vi "Main gScript UI.vi"() -> ()   [LabVIEW 2026]
uses:
  UI typedefs/gScript Controller Status.ctl
  gScript Interpreter/Type Definitions/Main Memory.ctl
  gScript Interpreter/Type Definitions/Memory Cell.ctl
  gScript Interpreter/Type Definitions/Memory Cell Type Enum.ctl
  gScript Interpreter/Type Definitions/Stack Frame.ctl
  gScript Interpreter/Type Definitions/Variable Table.ctl
  gScript Interpreter/Type Definitions/Variable.ctl
  Shared Components/Gantry Class/Type Definitions/Virtual Modes.ctl
  UI typedefs/gScript Controller Commands.ctl
  Shared Components/Gantry Class/Gantry.lvclass
  <instrlib>/Aerotech Automation1/Aerotech.Automation1.DotNet.dll
  gScript Interpreter/gScript Interpreter.lvclass
  Application Utilities/Console Log/Console Log.lvclass
  C:/Users/User/Desktop/pixel-gantry-control/Gantry/A3200/Bin/Aerotech.A3200.dll
  A3200/Bin/Aerotech.A3200.dll
  <instrlib>/Aerotech Automation1/Aerotech Automation1.lvlib
panel:
  out "Aerotech controller Ref":T2
  in  "Virtual Mode":bool=TRUE
  out "Command History idx":i32
  out "Abort Async Request":bool=TRUE
  in  "Tab Control":enum32{"Control", "Memory", "Command History"}(tab)
  in  "Load Project":bool
  out "Line Indicator":string
  out "version":string
  out "Script Path":path
  in  "ESTOP":bool
  in  "Execute":bool
  in  "Command Input":string
  out "Status":T3
  in  "Abort Script":bool
  in  "EXIT":bool
  in  "Pause Script":bool
  in  "Run Script":bool
  in  "Load Script":bool
  in  "Script Input":string
  in  "Save Script":bool
  out "Console":string
  in  "Variable Table":T4[](array[typedef])
  in  "Main Memory":T9
  in  "Memory Size":i32=256
  out "Command History":string[](array[string])
  # "Documentation:  https://github.com/CUASAS/pixel-gantry-control/blob/master/Gantry/gScript%20Application/gScript%20Documentation.md"
  # "Command Input >"
  # "Stack Index"
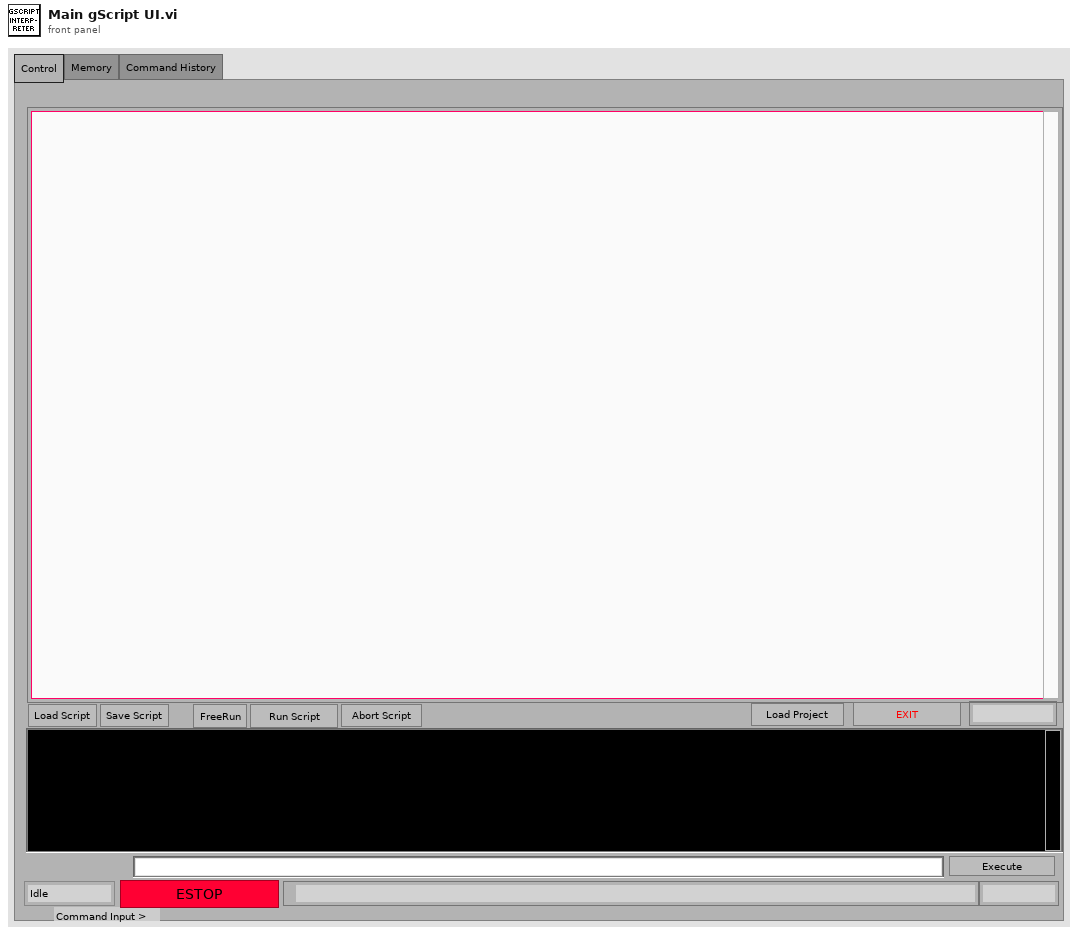
[diagram p1: front panel]
types:
  T1 = typedef "Virtual Modes.ctl" = enum16{"Nonvirtual", "Virtual"}
  T2 = cluster{"Controller Ref":variant, "Virtual Mode":T1}
  T3 = typedef "gScript Controller Status.ctl" = enum16{"Idle", "Running", "Paused"}
  T4 = typedef "Stack Frame.ctl" = cluster{"Variable Table":T5, "Return Pointer":i32, "Return Bindings":string[]}
  T5 = typedef "Variable Table.ctl" = T6[]
  T6 = typedef "Variable.ctl" = cluster{"Variable Name":string, "Memory Cell":T7}
  T7 = typedef "Memory Cell.ctl" = cluster{"type":T8, "x":dbl, "y":dbl, "z":dbl, "w":dbl}
  T8 = typedef "Memory Cell Type Enum.ctl" = enum16{"integer", "float", "vector", "rotation"}
  T9 = typedef "Main Memory.ctl" = T7[]
  T10 = typedef "gScript Controller Commands.ctl" = enum16{"Initialize", "Run Script", "Abort Script", "Exit", "Load Script", "Save Script", "Run Command", "ESTOP Pressed", "Quicksave", "Load Project"}
  T11 = enum8{"Enabled", "Disabled", "Disabled and Grayed Out"}
  T12 = cluster{"Shift":bool, "Ctrl":bool, "Alt":bool, "Cmd":bool, "Opt":bool}
  T13 = enum16{"open", "replace", "create", "open or create", "replace or create", "replace or create with confirmation"}
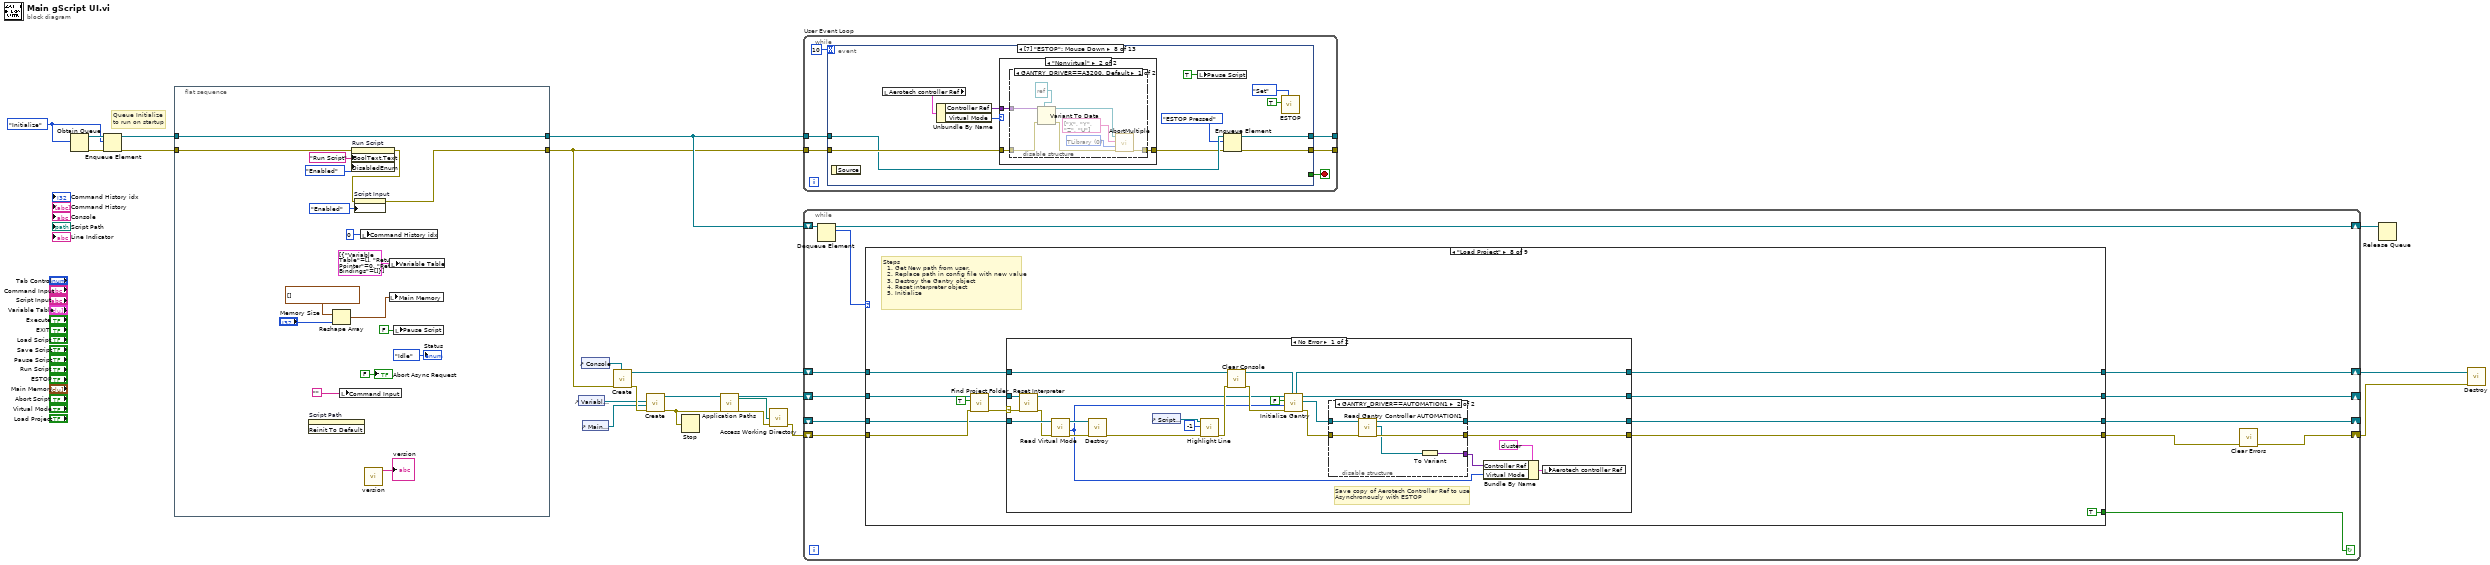
[diagram p0: block diagram]
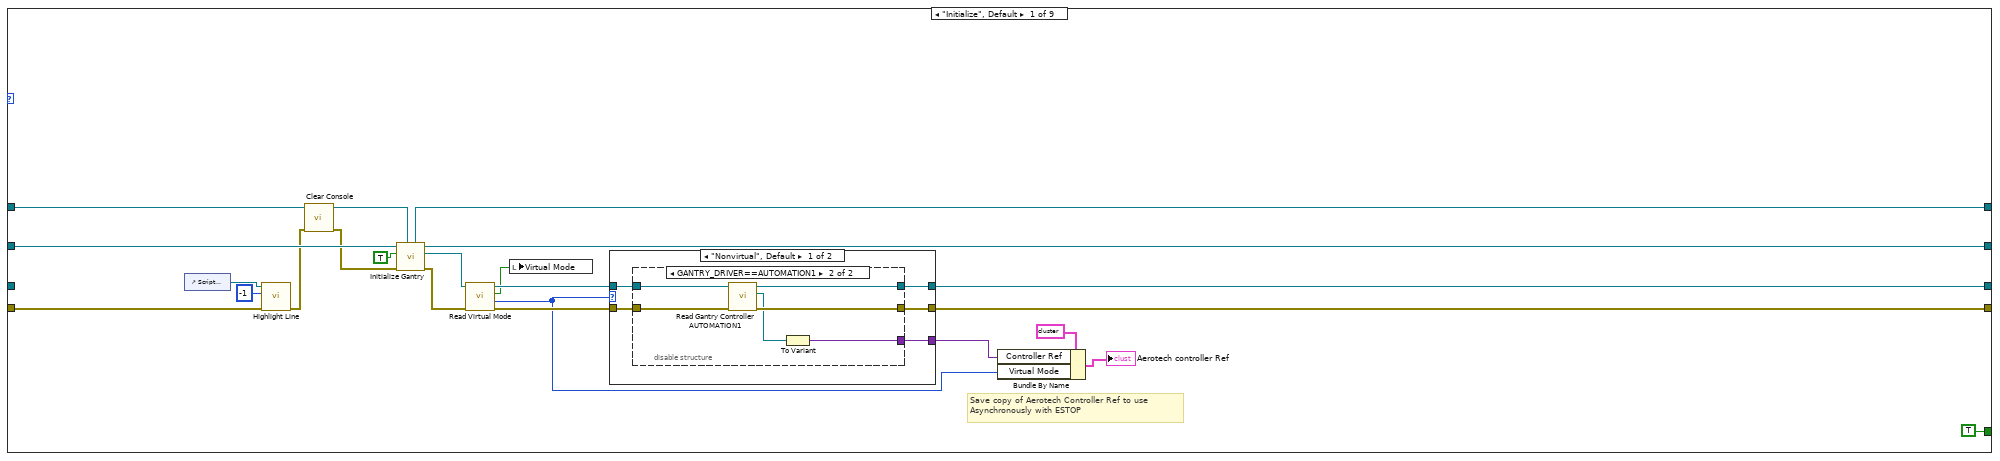
[diagram p2: hidden frame]
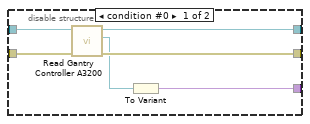
[diagram p3: hidden frame]
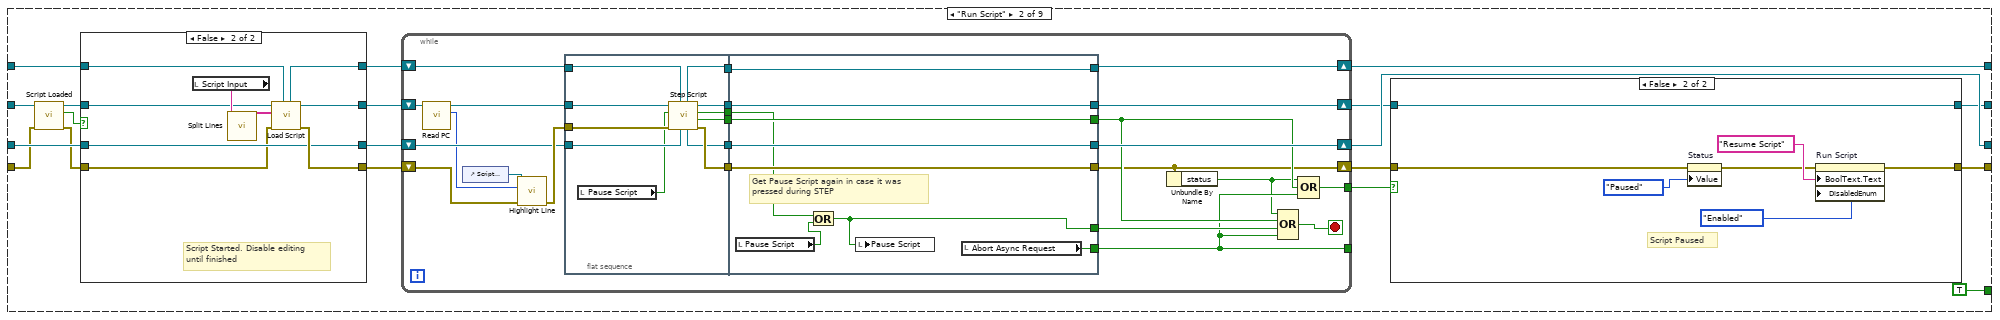
[diagram p5: hidden frame]
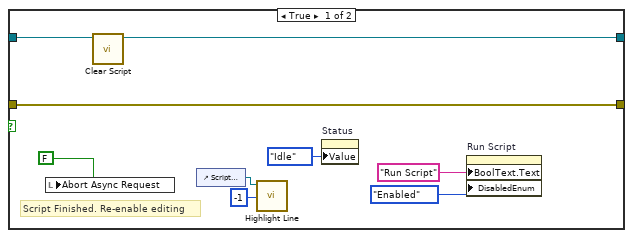
[diagram p7: hidden frame]
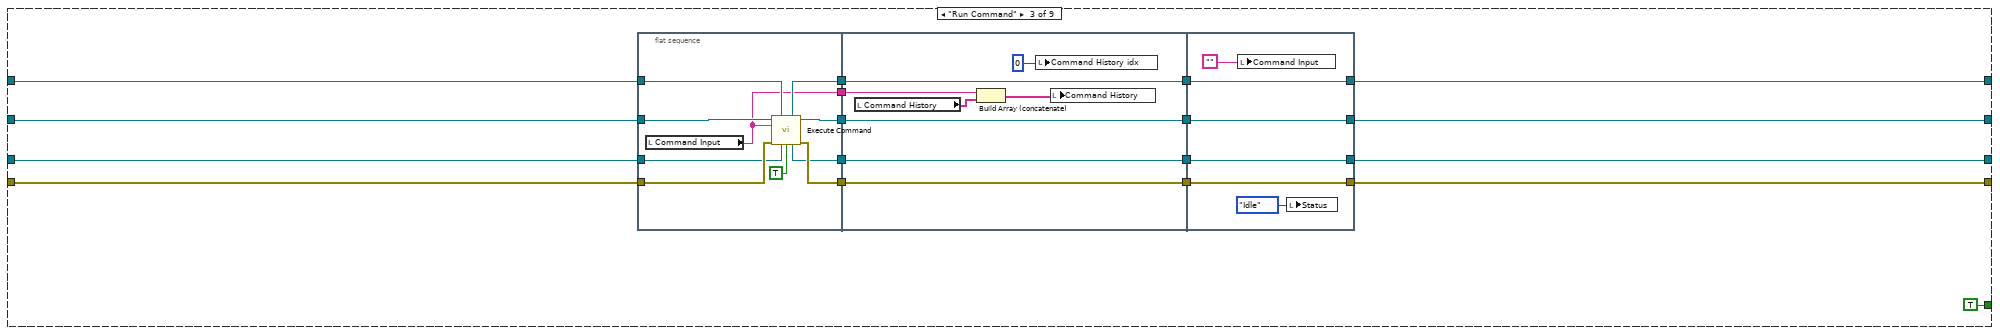
[diagram p8: hidden frame]
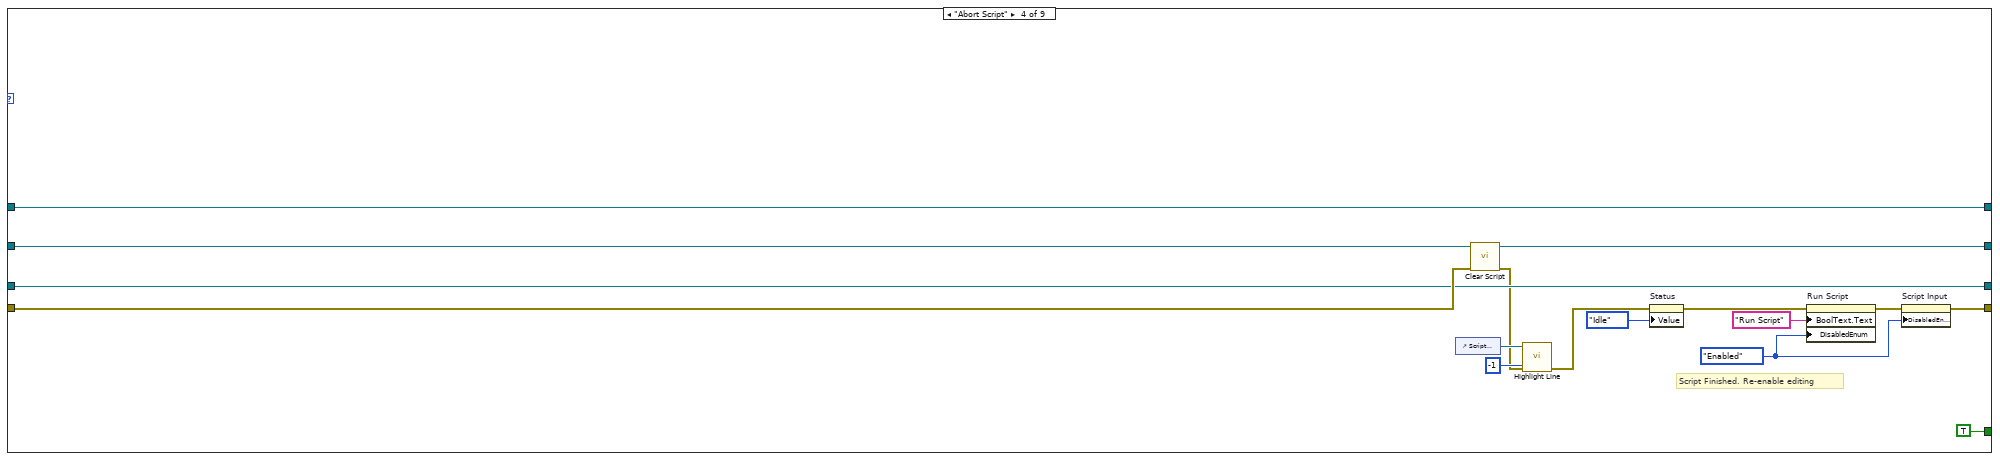
[diagram p9: hidden frame]
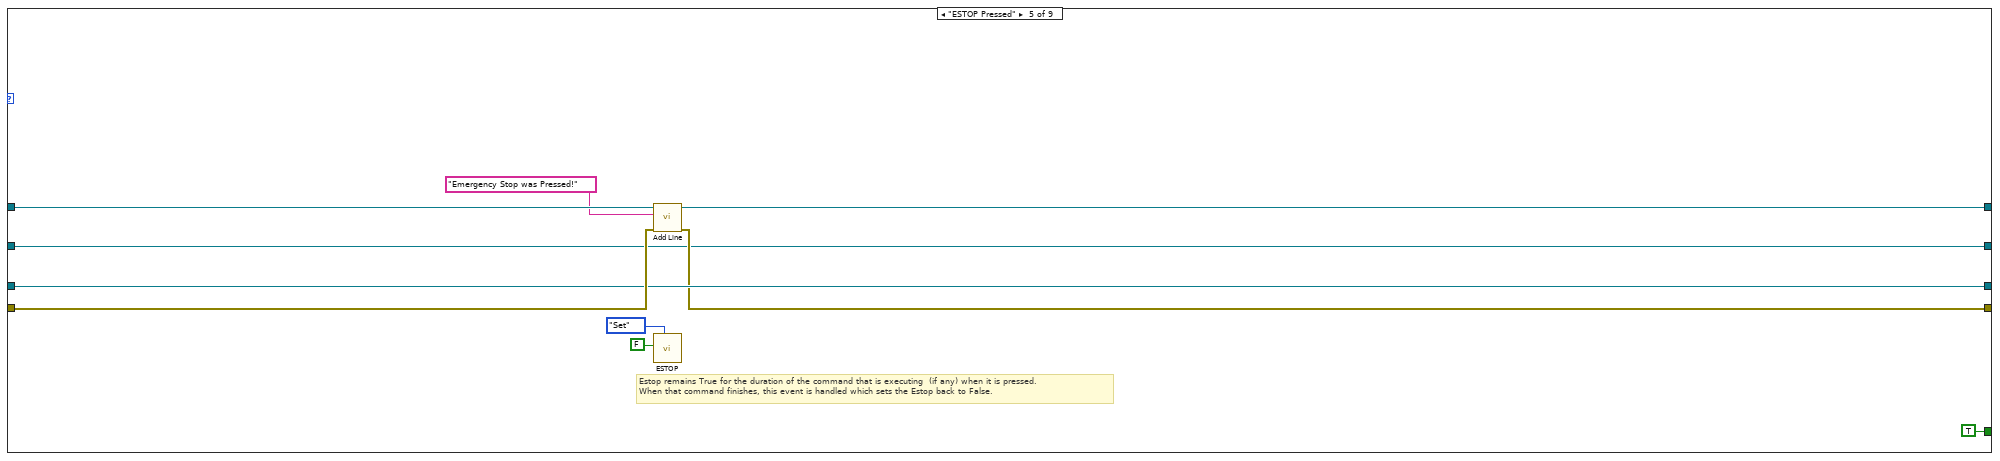
[diagram p10: hidden frame]
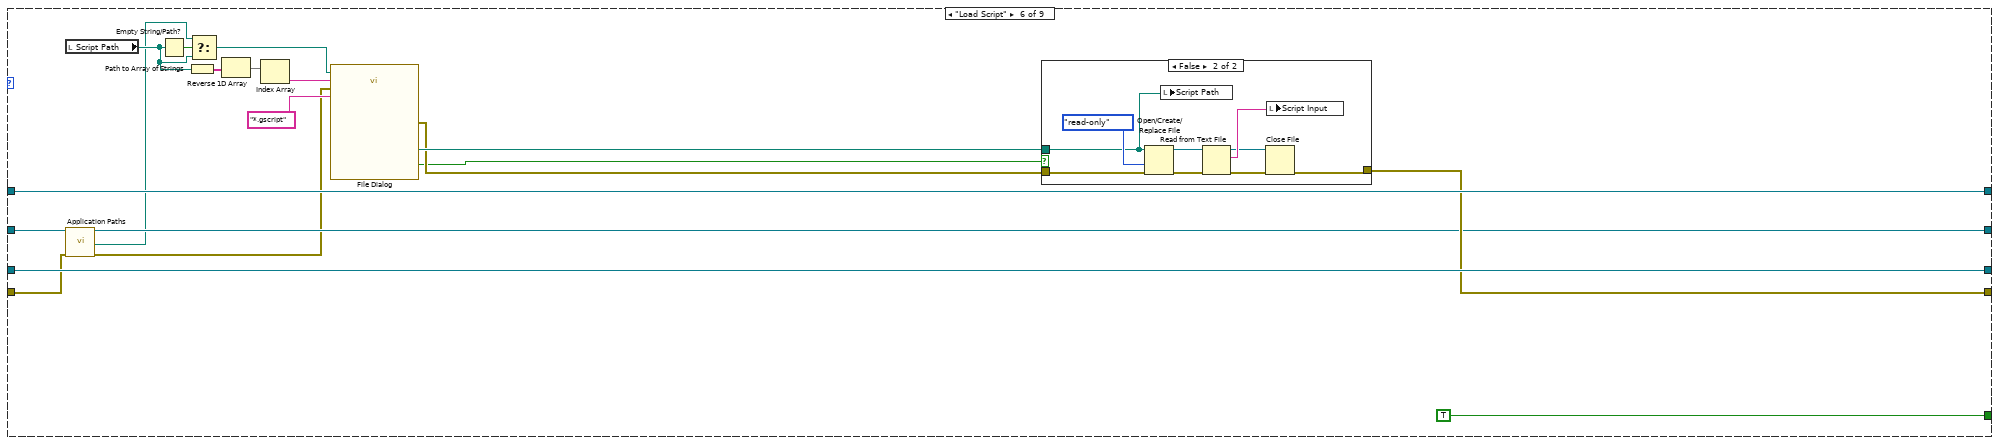
[diagram p11: hidden frame]
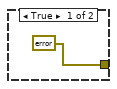
[diagram p12: hidden frame]
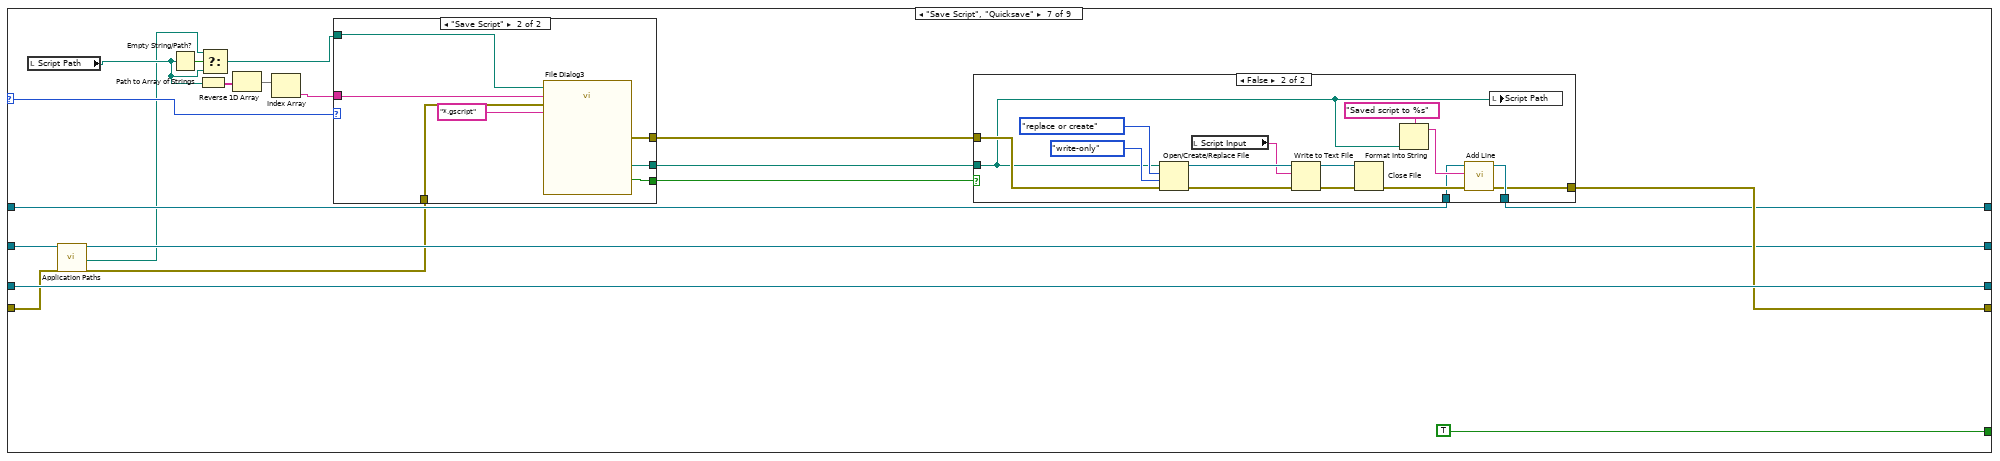
[diagram p13: hidden frame]
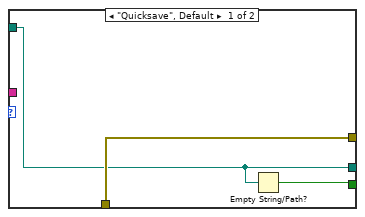
[diagram p14: hidden frame]
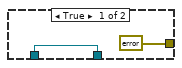
[diagram p15: hidden frame]
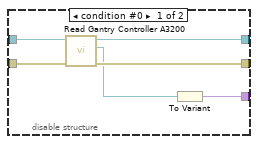
[diagram p16: hidden frame]
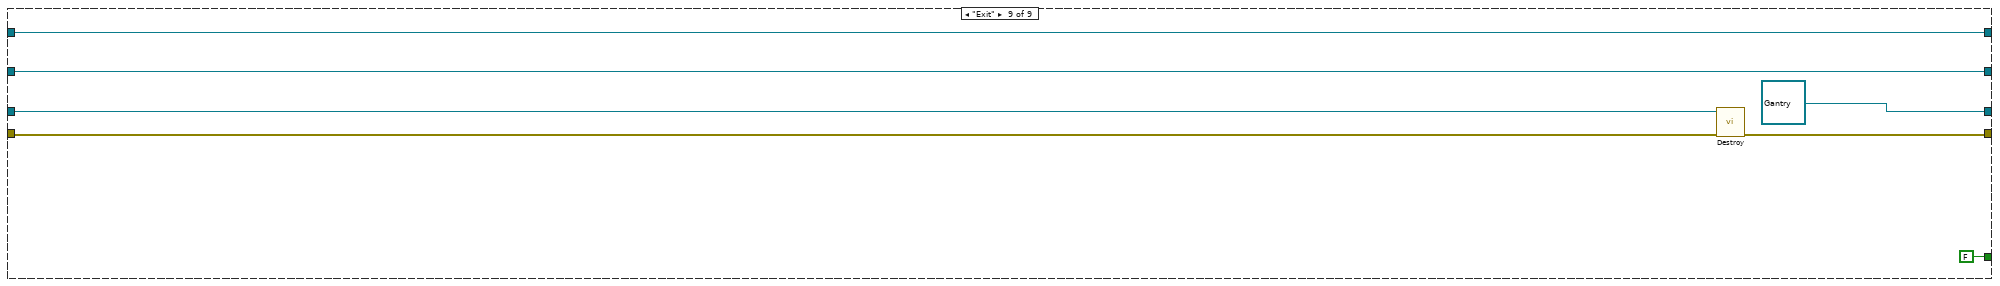
[diagram p18: hidden frame]
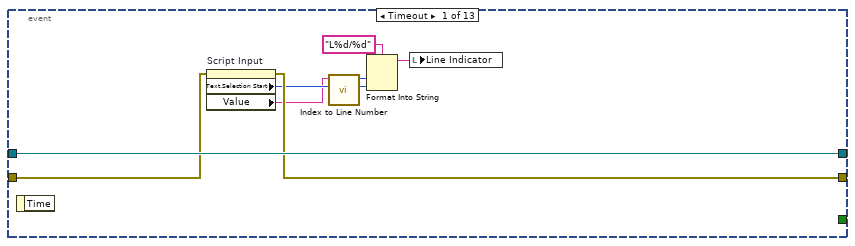
[diagram p19: hidden frame]
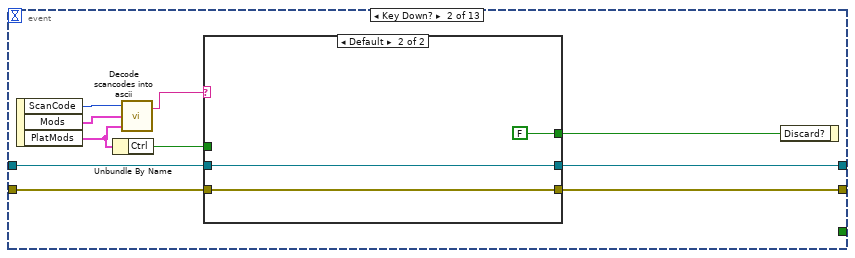
[diagram p20: hidden frame]
diagram:
  w18 = gScript_Controller_Commands."Initialize"
  # "Queue Initialize \nto run on startup"
  n1 = Obtain Queue(element data type=w18) -> (queue out=w20:refnum<queue>, error out=w19:errorcluster)  [unwired: 4 in, 1 out]
  n2 = Enqueue Element(queue=w20, element=w18, error in (no error)=w19) -> (queue out=w14:refnum<queue>, error out=w12:errorcluster)  [unwired: 1 in, 1 out]
  n3 = flat-sequence {
    tunnel: w14 -> [w38]
    tunnel: [w38] -> w13
    tunnel: w12 -> [w34]
    tunnel: [w31] -> w11
    frame #0 {
      n4 = invoke on="Script Path" class="Path" method="Reinit To Default"() -> ()  [unwired: 3 in, 3 out]
      n5 = Reshape Array(T7[] [] ("Main Memory"), "Memory Size") -> (w26:T7[])
      n6 = local write "Command Input"("") -> ()
      n7 = property on="Run Script" class="Bool (strict)"(error in=w34, "BoolText.Text"="Run Script" ("Boolean Text.Text"), "DisabledEnum"=T11."Enabled" ("Disabled")) -> (error out=w32:errorcluster)  [unwired: 1 in, 1 out]
      n8 = property on="Script Input" class="Str"(error in=w32, "DisabledEnum"=T11."Enabled" ("Disabled")) -> (error out=w31:errorcluster)  [unwired: 1 in, 1 out]
      n9 = local write "Command History idx"(0 ("Command History idx")) -> ()
      n10 = call "version.vi"() -> ("Version"=→"version":string)  [unwired: 3 in]
      n11 = local write "Main Memory"(w26) -> ()
      n12 = local write "Variable Table"(T4[] [{"Variable Table"=[], "Return Pointer"=0, "Return Bindings"=[]}] ("Variable Table")) -> ()
      n13 = local write "Pause Script"(FALSE ("Pause Script")) -> ()
      "Status" <- gScript_Controller_Status."Idle" ("Status")
      "Abort Async Request" <- FALSE ("Abort Requested")
    }
  }
  n14 = control-ref of="Variable Table"() -> (w7:refnum<vi>)
  n15 = control-ref of="Console"() -> (w21:refnum<vi>)
  n16 = control-ref of="Main Memory"() -> (w9:refnum<vi>)
  n17 = call "Create.vi"("Console"=w21, "error in"=w11) -> ("error out"=w15:errorcluster, "Console Log out"=w17:refnum<class "Console Log.lvclass">)  [unwired: 8 in]
  n18 = call "Create.vi"("error in (no error)"=w15, "Main Memory Ref"=w9, "Variable Table Ref"=w7) -> ("error out"=w1:errorcluster, "gScript Interpreter out"=w6:refnum<class "gScript Interpreter.lvclass">)  [unwired: 7 in]
  n19 = Stop(stop? (T)=w1) -> ()
  n20 = call "Application Paths.vi"("gScript Interpreter in"=w6, "error in (no error)"=w1) -> ("gScript Interpreter out"=w3:refnum<class "gScript Interpreter.lvclass">, "Project Path"=w2:path, "error out"=w5:errorcluster)  [unwired: 12 in, 3 out]
  n21 = call "Access Working Directory.vi"("error in (no error)"=w5, "Set Directory"=w2) -> ("error out"=w4:errorcluster)  [unwired: 2 in, 1 out]
  n22 = while "User Event Loop" {
    tunnel: w13 -> [w39]
    tunnel: [w42] -> _
    tunnel: w11 -> [w41]
    tunnel: [w40] -> _
    stop <- w43 stop-if-true
    n23 = event shown="[7] \"ESTOP\": Mouse Down" {
      selector: _ -> [_ _ _ _ _ _ _ _ _ _ _ _ _]
      dyn-events: _ -> [_ _ _ _ _ _ _ _ _ _ _ _ _]
      timeout: 10 -> [_ _ _ _ _ _ _ _ _ _ _ _ _]
      tunnel: [_ _ _ _ _ _ _ _ _ _ TRUE ("T button?") _ TRUE ("T button?")] -> w43
      tunnel: w39 -> [w53 w58 w85 w122 w138 w180 w202 w221 w247 w260 w272 w286 w292]
      tunnel: [w53 w56 w83 w120 w136 w177 w201 w218 w244 w258 w277 w284 w290] -> w42
      tunnel: w41 -> [w52 w57 w84 w121 w137 w179 w200 w223 w246 w259 w271 w285 w291]
      tunnel: [w51 w55 w82 w119 w135 w178 w199 w219 w243 w257 w276 w283 w289] -> w40
      event Timeout {
        n24 = event-data() -> ()  [unwired: 1 in, 1 out]
        n25 = property on="Script Input" class="Str"(error in=w52) -> (error out=w51:errorcluster, "Text.Selection Start"=w50:u32, "Value"=w49:string)  [unwired: 1 in, 1 out]
        n26 = call "Index to Line Number.vi"("Index"=w50, "Text"=w49) -> ("Line Count"=w45:u32, "Line Number"=w47:u32)  [unwired: 8 in]
        n27 = Format Into String(format string="L%d/%d", w47, w45) -> (resulting string=w46:string)  [unwired: 2 in, 1 out]
        n28 = local write "Line Indicator"(w46) -> ()
      }
      event Key Down? {
        n29 = event-data() -> ("ScanCode"=w63:i16, "Mods"=w61:cluster{"Num Pad":bool, "Menu Key":bool}, "PlatMods"=w60:T12)  [unwired: 1 in]
        n30 = Unbundle By Name(w60) -> ("Ctrl"=w59:bool)
        n31 = call "Decode scancodes into ascii.vi"("PlatMods"=w60, "Mods"=w61, "ScanCode"=w63) -> ("String"=w62:string)  [unwired: 1 out]
        n32 = case shown="Default" w62 {
          tunnel: w59 -> [w69 _]
          tunnel: w58 -> [w66 w81]
          tunnel: w57 -> [w68 w80]
          tunnel: [w65 w81] -> w56
          tunnel: [w67 w80] -> w55
          tunnel: [w64 FALSE] -> w54
          frame "s" {
            n33 = case shown="False" w69 {
              tunnel: w68 -> [w72 w77]
              tunnel: [w72 w76] -> w67
              tunnel: w66 -> [w71 w78]
              tunnel: [w71 w75] -> w65
              tunnel: [FALSE TRUE] -> w64
              frame False {
              }
              frame True {
                n34 = Enqueue Element(queue=w78, element=gScript_Controller_Commands."Quicksave", error in (no error)=w77) -> (queue out=w75:refnum<queue>, error out=w76:errorcluster)  [unwired: 1 in, 1 out]
              }
            }
          }
          frame Default {
          }
        }
        n35 = event-data("Discard?"=w54) -> ()  [unwired: 1 in, 1 out]
      }
      event "Script Input": Key Down? {
        n36 = event-data() -> ("ScanCode"=w90:i16, "Mods"=w89:cluster{"Num Pad":bool, "Menu Key":bool}, "PlatMods"=w88:T12)  [unwired: 1 in]
        n37 = local read "Status"() -> (w92:T3)
        n38 = call "Decode scancodes into ascii.vi"("PlatMods"=w88, "Mods"=w89, "ScanCode"=w90) -> ("Numeric"=w86:i16, "String"=w87:string)
        n39 = case shown="\"Idle\", Default" w92 {
          tunnel: [w98 TRUE] -> w91
          tunnel: w87 -> [w97 _]
          tunnel: w86 -> [_ _]
          tunnel: w85 -> [w96 w116]
          tunnel: w84 -> [w94 w115]
          tunnel: [w95 w116] -> w83
          tunnel: [w93 w115] -> w82
          frame "Idle", Default {
            n40 = case shown="\"tab\"" w97 {
              tunnel: [TRUE FALSE] -> w98
              tunnel: w96 -> [w99 w113]
              tunnel: [w99 w113] -> w95
              tunnel: w94 -> [w107 w112]
              tunnel: [w104 w112] -> w93
              frame "tab" {
                # "four spaces"
                n41 = control-ref of="Script Input"() -> (w110:refnum<vi>)
                n42 = property class="Str"(reference=w110, error in=w107) -> (reference out=w108:refnum<vi>, error out=w106:errorcluster, "Text.Selection End"=w102:u32, "Value"=w109:string)
                n43 = Add(x=w102, y=u32 4) -> (x+y=w100:u32)
                n44 = call "Insert Text.vi"("Insert String"="    ", "Insert Position"=w102, "Source String"=w109) -> ("Output String"=w105:string)
                n45 = property class="Str"(reference=w108, error in=w106, "Value"=w105, "Text.Selection End"=w100, "Text.Selection Start"=w100) -> (error out=w104:errorcluster)  [unwired: 1 out]
              }
              frame Default {
              }
            }
          }
          frame "Running", "Paused" {
            # "Disable editing the script while it is running"
          }
        }
        n46 = event-data("Discard?"=w91) -> ()  [unwired: 1 in, 1 out]
      }
      event "Execute": Value Change {
        n47 = event-data() -> ("NewVal"=w118:bool)  [unwired: 1 in]
        n48 = case shown="True" w118 {
          tunnel: w122 -> [w123 w130]
          tunnel: w121 -> [w124 w127]
          tunnel: [w123 w129] -> w120
          tunnel: [w124 w126] -> w119
          frame False {
          }
          frame True {
            n49 = Enqueue Element(queue=w130, element=gScript_Controller_Commands."Run Command", error in (no error)=w127) -> (queue out=w129:refnum<queue>, error out=w126:errorcluster)  [unwired: 1 in, 1 out]
            n50 = local write "Status"(gScript_Controller_Status."Running" ("Status")) -> ()
          }
        }
      }
      event "Command Input": Key Down {
        n51 = event-data() -> ("ScanCode"=w134:i16, "Mods"=w133:cluster{"Num Pad":bool, "Menu Key":bool}, "PlatMods"=w132:T12)  [unwired: 1 in]
        n52 = call "Decode scancodes into ascii.vi"("PlatMods"=w132, "Mods"=w133, "ScanCode"=w134) -> ("String"=w131:string)  [unwired: 1 out]
        n53 = case shown="\"UP\"" w131 {
          tunnel: w138 -> [w144 w153 w154 w163]
          tunnel: w137 -> [w143 w152 w155 w161]
          tunnel: [w144 w153 w154 w162] -> w136
          tunnel: [w143 w152 w155 w160] -> w135
          frame "UP" {
            n54 = local read "Command History idx"() -> (w140:i32)
            n55 = local read "Command History"() -> (w142:string[])
            n56 = Index Array(array=w142, index=w140) -> (element=w141:string)
            n57 = Increment(x=w140) -> (x+1=w139:i32)
            n58 = local write "Command Input"(w141) -> ()
            n59 = local write "Command History idx"(w139) -> ()
          }
          frame "DOWN" {
            n60 = local read "Command History idx"() -> (w149:i32)
            n61 = local read "Command History"() -> (w150:string[])
            n62 = Decrement(x=w149) -> (x-1=w148:i32)
            n63 = In Range and Coerce(upper limit=1000 ("lower limit"), x=w148, lower limit=0) -> (coerced(x)=w147:i32)  [unwired: 1 out]
            n64 = Index Array(array=w150, index=w147) -> (element=w146:string)
            n65 = local write "Command Input"(w146) -> ()
            n66 = local write "Command History idx"(w147) -> ()
          }
          frame Default {
          }
          frame "Enter" {
            n67 = flat-sequence {
              tunnel: w163 -> [w166]
              tunnel: w161 -> [w167]
              tunnel: [w167] -> w159
              tunnel: [w166] -> w158
              tunnel: w159 -> [w168]
              tunnel: w158 -> [w170]
              tunnel: [w172] -> w157
              tunnel: [w171] -> w156
              tunnel: [w174] -> w160
              tunnel: [w175] -> w162
              tunnel: w157 -> [w175]
              tunnel: w156 -> [w174]
              frame #0 {
                # "Does not work without this pause"
                n68 = local write "Status"(gScript_Controller_Status."Running" ("Status")) -> ()
                n69 = Wait (ms)(milliseconds to wait=u32 100) -> ()  [unwired: 1 out]
              }
              frame #1 {
                n70 = Enqueue Element(queue=w170, element=gScript_Controller_Commands."Run Command", error in (no error)=w168) -> (queue out=w172:refnum<queue>, error out=w171:errorcluster)  [unwired: 1 in, 1 out]
              }
              frame #2 {
                n71 = property on="Command Input" class="Str"("Key Focus"=TRUE) -> ()  [unwired: 2 in, 2 out]
              }
            }
          }
        }
      }
      event "Run Script": Mouse Up {
        n72 = event-data() -> ()  [unwired: 1 in, 1 out]
        n73 = local read "Status"() -> (w176:T3)
        n74 = case shown="\"Idle\"" w176 {
          tunnel: w180 -> [w182 w190 w197]
          tunnel: w179 -> [w181 w189 w196]
          tunnel: [w181 w188 w193] -> w178
          tunnel: [w182 w187 w194] -> w177
          frame "Running" {
          }
          frame "Idle" {
            n75 = Enqueue Element(queue=w190, element=gScript_Controller_Commands."Run Script", error in (no error)=w189) -> (queue out=w187:refnum<queue>, error out=w188:errorcluster)  [unwired: 1 in, 1 out]
            n76 = property on="Run Script" class="Bool (strict)"("BoolText.Text"="Running" ("Boolean Text.Text"), "DisabledEnum"=T11."Disabled and Grayed Out" ("Disabled")) -> ()  [unwired: 2 in, 2 out]
            n77 = local write "Status"(gScript_Controller_Status."Running" ("Status")) -> ()
          }
          frame "Paused" {
            n78 = Enqueue Element(queue=w197, element=gScript_Controller_Commands."Run Script", error in (no error)=w196) -> (queue out=w194:refnum<queue>, error out=w193:errorcluster)  [unwired: 1 in, 1 out]
            n79 = property on="Run Script" class="Bool (strict)"("BoolText.Text"="Running" ("Boolean Text.Text"), "DisabledEnum"=T11."Disabled and Grayed Out" ("Disabled")) -> ()  [unwired: 2 in, 2 out]
            n80 = local write "Status"(gScript_Controller_Status."Running" ("Status")) -> ()
          }
        }
      }
      event "Abort Script": Mouse Up {
        n81 = event-data() -> ()  [unwired: 1 in, 1 out]
        n82 = local read "Status"() -> (w203:T3)
        n83 = case shown="\"Idle\", \"Paused\"" w203 {
          tunnel: w202 -> [w205 w210]
          tunnel: [w205 w209] -> w201
          tunnel: w200 -> [w204 w208]
          tunnel: [w204 w207] -> w199
          frame "Running" {
            n84 = local write "Abort Async Request"(TRUE ("Abort Requested")) -> ()
          }
          frame "Idle", "Paused" {
            n85 = Enqueue Element(queue=w210, element=gScript_Controller_Commands."Abort Script", error in (no error)=w208) -> (queue out=w209:refnum<queue>, error out=w207:errorcluster)  [unwired: 1 in, 1 out]
          }
        }
      }
      event "ESTOP": Mouse Down {
        n86 = event-data() -> ()  [unwired: 1 in, 1 out]
        n87 = local read "Aerotech controller Ref"() -> (w214:T2)
        n88 = Unbundle By Name(w214) -> ("Controller Ref"=w213:variant, "Virtual Mode"=w212:T1)
        n89 = case shown="\"Nonvirtual\"" w212 {
          tunnel: w223 -> [w224 w225]
          tunnel: [w224 w227] -> w220
          tunnel: w213 -> [_ w226]
          frame "Virtual" {
          }
          frame "Nonvirtual" {
            n90 = disable-structure shown="GANTRY_DRIVER==A3200, Default" {
              disable-tunnel: [w233 w236] -> w227
              disable-tunnel: w226 -> [w231 w238]
              disable-tunnel: w225 -> [w229 w237]
              frame condition #0 {
                w234 = 0 items=["TLibrary", "T01", "T02", "T03", "T04", "T05", "T06", "T07", "T08", "T09", "T10", "T11", "T12", "T13", "T14", "T15", "T16", "T17", "T18", "T19", "T20", "T21", "T22", "T23", "T24", "T25", "T26", "T27", "T28", "T29", "T30", "T31"] ("taskId")
                n91 = Variant To Data(error in=w229, type=refnum<k24> refnum ("controller out"), Variant=w231) -> (data=w230:refnum<k24>, error out=w228:errorcluster)
                n92 = call "AbortMultiple.vi"("error in (no error)"=w228, "taskId"=w234, "axis names"=string[] ["X", "Y", "Z", "U"], "controller in"=w230) -> ("error out"=w233:errorcluster)  [unwired: 6 in, 1 out]
              }
              frame condition #1 (active) {
                n93 = Variant To Data(error in=w237, type=refnum<k24> refnum ("Controller Refnum out"), Variant=w238) -> (data=w241:refnum<k24>, error out=w240:errorcluster)
                n94 = call <instrlib>:"Abort.vi"("error in (no error)"=w240, "axisNames"=string[] ["X", "Y", "Z", "U"] ("axis names"), "Controller Refnum"=w241) -> ("error out"=w236:errorcluster)  [unwired: 7 in, 1 out]
              }
            }
          }
        }
        n95 = local write "Pause Script"(TRUE ("Pause Script")) -> ()
        n96 = Enqueue Element(queue=w221, element=gScript_Controller_Commands."ESTOP Pressed", error in (no error)=w220) -> (queue out=w218:refnum<queue>, error out=w219:errorcluster)  [unwired: 1 in, 1 out]
        n97 = call "ESTOP.vi"("Get/Set"=enum16{"Get", "Set"}."Set", "Value In"=TRUE) -> ()  [unwired: 9 in, 1 out]
      }
      event "Load Script": Mouse Up {
        n98 = event-data() -> ()  [unwired: 1 in, 1 out]
        n99 = local read "Status"() -> (w245:T3)
        n100 = case shown="\"Idle\", Default" w245 {
          tunnel: w247 -> [w252 w255]
          tunnel: w246 -> [w251 w254]
          tunnel: [w249 w255] -> w244
          tunnel: [w250 w254] -> w243
          frame "Idle", Default {
            n101 = Enqueue Element(queue=w252, element=gScript_Controller_Commands."Load Script", error in (no error)=w251) -> (queue out=w249:refnum<queue>, error out=w250:errorcluster)  [unwired: 1 in, 1 out]
          }
          frame "Running", "Paused" {
            n102 = One Button Dialog(message="Cannot Load while Script is Running or Paused\nAbort or finish running script first.") -> ()  [unwired: 1 in, 1 out]
          }
        }
      }
      event "Save Script": Mouse Up {
        n103 = event-data() -> ()  [unwired: 1 in, 1 out]
        n104 = local read "Status"() -> (w256:T3)
        n105 = case shown="\"Idle\", Default" w256 {
          tunnel: w260 -> [w265 w268]
          tunnel: w259 -> [w264 w267]
          tunnel: [w262 w268] -> w258
          tunnel: [w263 w267] -> w257
          frame "Idle", Default {
            n106 = Enqueue Element(queue=w265, element=gScript_Controller_Commands."Save Script", error in (no error)=w264) -> (queue out=w262:refnum<queue>, error out=w263:errorcluster)  [unwired: 1 in, 1 out]
          }
          frame "Running", "Paused" {
            n107 = One Button Dialog(message="Cannot Save while Script is Running or Paused\nAbort or finish running script first.") -> ()  [unwired: 1 in, 1 out]
          }
        }
      }
      event "EXIT": Mouse Up {
        n108 = event-data() -> ()  [unwired: 1 in, 1 out]
        n109 = local read "Status"() -> (w273:T3)
        n110 = case shown="Default" w273 {
          tunnel: w272 -> [w279 w281]
          tunnel: w271 -> [w278 w280]
          tunnel: [w279 w281] -> w270
          tunnel: [w278 w280] -> w269
          frame Default {
          }
          frame "Running" {
            n111 = local write "Abort Async Request"(TRUE ("Abort Async Request")) -> ()
          }
        }
        n112 = Enqueue Element(queue=w270, element=gScript_Controller_Commands."Exit", error in (no error)=w269) -> (queue out=w277:refnum<queue>, error out=w276:errorcluster)  [unwired: 1 in, 1 out]
      }
      event "Load Project": Mouse Up {
        n113 = event-data() -> ()  [unwired: 1 in, 1 out]
        n114 = Enqueue Element(queue=w286, element=gScript_Controller_Commands."Load Project", error in (no error)=w285) -> (queue out=w284:refnum<queue>, error out=w283:errorcluster)  [unwired: 1 in, 1 out]
      }
      event Panel Close? {
        n115 = event-data() -> ()  [unwired: 1 in, 1 out]
        n116 = Enqueue Element(queue=w292, element=gScript_Controller_Commands."Exit", error in (no error)=w291) -> (queue out=w290:refnum<queue>, error out=w289:errorcluster)  [unwired: 1 in, 1 out]
        n117 = event-data("Discard?"=TRUE) -> ()  [unwired: 1 in, 1 out]
      }
    }
  }
  n118 = while {
    shift-right: [w296] -> w16
    shift-left: w17 -> [w305]
    shift-right: [w299] -> _
    shift-left: w3 -> [w304]
    shift-right: [w302] -> _
    shift-left: _ -> [w303]
    shift-right: [w297] -> w8
    shift-left: w4 -> [w301]
    shift-right: [w298] -> w10
    shift-left: w13 -> [w307]
    stop <- w300 continue-if-true
    n119 = Dequeue Element(queue=w307) -> (queue out=w298:refnum<queue>, element=w306:T10)  [unwired: 2 in, 2 out]
    n120 = case shown="\"Load Project\"" w306 {
      selector: w306 -> [_ _ _ _ _ _ w552 _ _]
      tunnel: w305 -> [w323 w359 w457 w490 w509 w526 w551 w592 w643]
      tunnel: w304 -> [w325 w357 w459 w493 w502 w514 w543 w597 w644]
      tunnel: w303 -> [_ w361 w453 w487 w506 w528 w558 w587 w641]
      tunnel: [w327 w352 w452 w487 w506 w528 w558 w590 refnum<class "Gantry.lvclass"> refnum ("Gantry Out")] -> w302
      tunnel: w301 -> [w326 w355 w455 w492 w507 w512 w541 w595 w642]
      tunnel: [w312 w363 w454 w489 w505 w522 w556 w588 w640] -> w295
      tunnel: [TRUE TRUE TRUE TRUE TRUE TRUE TRUE TRUE FALSE] -> w300
      tunnel: [w318 w364 w456 w490 w503 w526 w550 w591 w643] -> w296
      tunnel: [w319 w350 w458 w491 w502 w513 w542 w589 w644] -> w299
      frame "Initialize", Default {
        # "Save copy of Aerotech Controller Ref to use\nAsynchronously with ESTOP"
        n121 = control-ref of="Script Input"() -> (w329:refnum<vi>)
        n122 = call "Highlight Line.vi"("error in (no error)"=w326, "Line Number"=-1, "String Field In"=w329) -> ("error out"=w321:errorcluster)  [unwired: 7 in, 1 out]
        n123 = call "Clear Console.vi"("error in (no error)"=w321, "Console Log in"=w323) -> ("error out"=w320:errorcluster, "Console Log out"=w322:refnum<class "Console Log.lvclass">)  [unwired: 8 in]
        n124 = call "Initialize Gantry.vi"("Console Log in"=w322, "error in (no error)"=w320, "Prompt for Virtual Mode"=TRUE, "gScript Interpreter in"=w325) -> ("error out"=w314:errorcluster, "Gantry out"=w317:refnum<class "Gantry.lvclass">, "gScript Interpreter out"=w319:refnum<class "gScript Interpreter.lvclass">, "Console Log out"=w318:refnum<class "Console Log.lvclass">)  [unwired: 4 in]
        n125 = call-dynamic "Read Virtual Mode.vi"("error in (no error)"=w314, "Gantry in"=w317) -> ("error out"=w313:errorcluster, "Virtual Mode"=w309:T1, "Is Virtual"=w315:bool, "Gantry out"=w316:refnum<class "Gantry.lvclass">)  [unwired: 6 in]
        n126 = local write "Virtual Mode"(w315) -> ()
        n127 = case shown="\"Nonvirtual\", Default" w309 {
          tunnel: [w333 w349] -> w327
          tunnel: w316 -> [w335 w349]
          tunnel: w313 -> [w334 w348]
          tunnel: [w332 w348] -> w312
          tunnel: [w331 _] -> w311
          frame "Nonvirtual", Default {
            n128 = disable-structure shown="GANTRY_DRIVER==AUTOMATION1" {
              disable-tunnel: w335 -> [w341 w347]
              disable-tunnel: w334 -> [w339 w346]
              disable-tunnel: [w340 w344] -> w333
              disable-tunnel: [w338 w345] -> w332
              disable-tunnel: [w336 w343] -> w331
              frame condition #0 {
                n129 = call "Read Gantry Controller A3200.vi"("error in (no error)"=w339, "Gantry in"=w341) -> ("error out"=w338:errorcluster, "A3200 controller out"=w337:refnum<k24>, "Gantry out"=w340:refnum<class "Gantry.lvclass">)  [unwired: 7 in]
                n130 = To Variant(anything=w337) -> (Variant=w336:variant)
              }
              frame condition #1 (active) {
                n131 = call "Read Gantry Controller AUTOMATION1.vi"("error in (no error)"=w346, "Gantry in"=w347) -> ("error out"=w345:errorcluster, "Controller AUTOMATION1"=w342:refnum<k24>, "Gantry out"=w344:refnum<class "Gantry.lvclass">)  [unwired: 7 in]
                n132 = To Variant(anything=w342) -> (Variant=w343:variant)
              }
            }
          }
          frame "Virtual" {
          }
        }
        n133 = Bundle By Name(cluster=T2 {"Controller Ref"=variant, "Virtual Mode"=enum."Nonvirtual"} ("Aerotech controller Ref"), "Controller Ref"=w311, "Virtual Mode"=w309) -> (→"Aerotech controller Ref":T2)
      }
      frame "Run Script" {
        n134 = call-dynamic "Script Loaded.vi"("error in (no error)"=w355, "gScript Interpreter in"=w357) -> ("error out"=w354:errorcluster, "Script Loaded?"=w353:bool, "gScript Interpreter out"=w356:refnum<class "gScript Interpreter.lvclass">)  [unwired: 7 in]
        n135 = case shown="False" w353 {
          tunnel: w356 -> [w372 w380]
          tunnel: [w372 w379] -> w367
          tunnel: w354 -> [w369 w375]
          tunnel: [w369 w377] -> w366
          tunnel: w361 -> [w370 w376]
          tunnel: [w370 w376] -> w360
          tunnel: w359 -> [w371 w374]
          tunnel: [w371 w373] -> w358
          frame True {
          }
          frame False {
            # "Script Started. Disable editing\nuntil finished"
            n136 = local read "Script Input"() -> (w381:string)
            n137 = call "Split Lines.vi"("String In"=w381) -> ("Lines Out"=w378:string[])  [unwired: 10 in]
            n138 = call-dynamic "Load Script.vi"("Console Log in"=w374, "error in (no error)"=w375, "Commands In"=w378, "gScript Interpreter in"=w380) -> ("error out"=w377:errorcluster, "gScript Interpreter out"=w379:refnum<class "gScript Interpreter.lvclass">, "Console Log out"=w373:refnum<class "Console Log.lvclass">)  [unwired: 5 in]
          }
        }
        n139 = while {
          shift-right: [w405] -> w365
          shift-left: w366 -> [w421]
          shift-right: [w418] -> w352
          shift-left: w360 -> [w419]
          shift-right: [w414] -> w351
          shift-left: w367 -> [w413]
          shift-right: [w415] -> w364
          shift-left: w358 -> [w416]
          tunnel: [w407] -> w362
          tunnel: [w406] -> _
          stop <- w409 stop-if-true
          n140 = call-dynamic "Read PC.vi"("gScript Interpreter in"=w413) -> ("PC"=w411:i32, "gScript Interpreter out"=w412:refnum<class "gScript Interpreter.lvclass">)  [unwired: 8 in, 1 out]
          n141 = control-ref of="Script Input"() -> (w417:refnum<vi>)
          n142 = call "Highlight Line.vi"("error in (no error)"=w421, "Line Number"=w411, "String Field In"=w417) -> ("error out"=w420:errorcluster)  [unwired: 7 in, 1 out]
          n143 = flat-sequence {
            tunnel: w420 -> [w432]
            tunnel: w419 -> [w430]
            tunnel: w416 -> [w428]
            tunnel: w412 -> [w425]
            tunnel: [w431] -> w403
            tunnel: [w429] -> w402
            tunnel: [w427] -> w401
            tunnel: [w426] -> w400
            tunnel: [w424] -> w399
            tunnel: [w422] -> w398
            tunnel: [w436] -> w406
            tunnel: [w437] -> w408
            tunnel: [w435] -> w410
            tunnel: [w438] -> w414
            tunnel: [w439] -> w415
            tunnel: [w440] -> w418
            tunnel: [w441] -> w405
            tunnel: w398 -> [w433]
            tunnel: w399 -> [w437]
            tunnel: w400 -> [w438]
            tunnel: w401 -> [w439]
            tunnel: w402 -> [w440]
            tunnel: w403 -> [w441]
            frame #0 {
              n144 = local read "Pause Script"() -> (w423:bool)
              n145 = call-dynamic "Step Script.vi"("Gantry In"=w430, "Console Log In"=w428, "error in (no error)"=w432, "Pause in"=w423, "gScript Interpreter in"=w425) -> ("error out"=w431:errorcluster, "Finished"=w424:bool, "Pause out"=w422:bool, "gScript Interpreter out"=w426:refnum<class "gScript Interpreter.lvclass">, "Gantry Out"=w429:refnum<class "Gantry.lvclass">, "Console Log Out"=w427:refnum<class "Console Log.lvclass">)  [unwired: 1 in]
            }
            frame #1 {
              # "Get Pause Script again in case it was\npressed during STEP"
              n146 = local read "Pause Script"() -> (w434:bool)
              n147 = Or(x=w433, y=w434) -> (x .or. y?=w435:bool)
              n148 = local write "Pause Script"(w435) -> ()
              n149 = local read "Abort Async Request"() -> (w436:bool)
            }
          }
          n150 = Unbundle By Name(w405) -> ("status"=w404:bool)
          n151 = Compound Arithmetic op=OR(w404, w408, w410, w406) -> (w409:bool)
          n152 = Compound Arithmetic op=OR(w404, w408, w406) -> (w407:bool)
        }
        n153 = case shown="False" w362 {
          tunnel: w365 -> [w382 w397]
          tunnel: [w382 w392] -> w363
          tunnel: w351 -> [w385 w391]
          tunnel: [w384 w391] -> w350
          frame True {
            # "Script Finished. Re-enable editing"
            n154 = local write "Abort Async Request"(FALSE ("Abort Requested")) -> ()
            n155 = call-dynamic "Clear Script.vi"("gScript Interpreter in"=w385) -> ("gScript Interpreter out"=w384:refnum<class "gScript Interpreter.lvclass">)  [unwired: 9 in, 1 out]
            n156 = control-ref of="Script Input"() -> (w388:refnum<vi>)
            n157 = call "Highlight Line.vi"("Line Number"=-1, "String Field In"=w388) -> ()  [unwired: 8 in, 2 out]
            n158 = property on="Status" class="Enum (strict)"("Value"=gScript_Controller_Status."Idle" ("Status")) -> ()  [unwired: 2 in, 2 out]
            n159 = property on="Run Script" class="Bool (strict)"("BoolText.Text"="Run Script" ("Boolean Text.Text"), "DisabledEnum"=T11."Enabled" ("Disabled")) -> ()  [unwired: 2 in, 2 out]
          }
          frame False {
            # "Script Paused"
            n160 = property on="Status" class="Enum (strict)"(error in=w397, "Value"=gScript_Controller_Status."Paused" ("Status")) -> (error out=w393:errorcluster)  [unwired: 1 in, 1 out]
            n161 = property on="Run Script" class="Bool (strict)"(error in=w393, "BoolText.Text"="Resume Script" ("Boolean Text.Text"), "DisabledEnum"=T11."Enabled" ("Disabled")) -> (error out=w392:errorcluster)  [unwired: 1 in, 1 out]
          }
        }
      }
      frame "Run Command" {
        n162 = flat-sequence {
          tunnel: w459 -> [w469]
          tunnel: w457 -> [w467]
          tunnel: w455 -> [w465]
          tunnel: w453 -> [w461]
          tunnel: [w468] -> w450
          tunnel: [w466] -> w448
          tunnel: [w464] -> w446
          tunnel: [w463] -> w444
          tunnel: [w462] -> w442
          tunnel: w450 -> [w477]
          tunnel: [w477] -> w449
          tunnel: w448 -> [w476]
          tunnel: [w476] -> w447
          tunnel: w446 -> [w475]
          tunnel: [w475] -> w445
          tunnel: w444 -> [w474]
          tunnel: [w474] -> w443
          tunnel: w442 -> [w472]
          tunnel: [w480] -> w452
          tunnel: [w481] -> w454
          tunnel: [w482] -> w456
          tunnel: [w483] -> w458
          tunnel: w449 -> [w483]
          tunnel: w447 -> [w482]
          tunnel: w445 -> [w481]
          tunnel: w443 -> [w480]
          frame #0 {
            n163 = local read "Command Input"() -> (w462:string)
            n164 = call-dynamic "Execute Command.vi"("gScript Interpreter in"=w469, "Console Log In"=w467, "Command"=w462, "error in (no error)"=w465, "Gantry In"=w461, "Is Interactive"=TRUE) -> ("Console Log Out"=w466:refnum<class "Console Log.lvclass">, "gScript Interpreter out"=w468:refnum<class "gScript Interpreter.lvclass">, "Gantry Out"=w463:refnum<class "Gantry.lvclass">, "error out"=w464:errorcluster)  [unwired: 4 in, 2 out]
          }
          frame #1 {
            n165 = local read "Command History"() -> (w473:string[])
            n166 = Build Array (concatenate)(w472, w473) -> (w471:string[])
            n167 = local write "Command History idx"(0 ("Command History idx")) -> ()
            n168 = local write "Command History"(w471) -> ()
          }
          frame #2 {
            n169 = local write "Command Input"("") -> ()
            n170 = local write "Status"(gScript_Controller_Status."Idle" ("Status")) -> ()
          }
        }
      }
      frame "Abort Script" {
        w494 = T11."Enabled" ("Disabled")
        # "Script Finished. Re-enable editing"
        n171 = control-ref of="Script Input"() -> (w488:refnum<vi>)
        n172 = call-dynamic "Clear Script.vi"("error in (no error)"=w492, "gScript Interpreter in"=w493) -> ("error out"=w485:errorcluster, "gScript Interpreter out"=w491:refnum<class "gScript Interpreter.lvclass">)  [unwired: 8 in]
        n173 = call "Highlight Line.vi"("error in (no error)"=w485, "Line Number"=-1, "String Field In"=w488) -> ("error out"=w484:errorcluster)  [unwired: 7 in, 1 out]
        n174 = property on="Status" class="Enum (strict)"(error in=w484, "Value"=gScript_Controller_Status."Idle" ("Status")) -> (error out=w497:errorcluster)  [unwired: 1 in, 1 out]
        n175 = property on="Run Script" class="Bool (strict)"(error in=w497, "BoolText.Text"="Run Script" ("Boolean Text.Text"), "DisabledEnum"=w494) -> (error out=w495:errorcluster)  [unwired: 1 in, 1 out]
        n176 = property on="Script Input" class="Str"(error in=w495, "DisabledEnum"=w494) -> (error out=w489:errorcluster)  [unwired: 1 in, 1 out]
      }
      frame "ESTOP Pressed" {
        # "Estop remains True for the duration of the command that is executing  (if any) when it is pressed.\nWhen that command finishes, this event is handled which sets the Estop back to False."
        n177 = call "Add Line.vi"("error in"=w507, "String"="Emergency Stop was Pressed!", "Console Log in"=w509) -> ("error out"=w505:errorcluster, "Console Log out"=w503:refnum<class "Console Log.lvclass">)  [unwired: 7 in]
        n178 = call "ESTOP.vi"("Get/Set"=enum16{"Get", "Set"}."Set", "Value In"=FALSE) -> ()  [unwired: 9 in, 1 out]
      }
      frame "Load Script" {
        n179 = local read "Script Path"() -> (w516:path)
        n180 = call "Application Paths.vi"("gScript Interpreter in"=w514, "error in (no error)"=w512) -> ("gScript Interpreter out"=w513:refnum<class "gScript Interpreter.lvclass">, "Scripts Path"=w510:path, "error out"=w511:errorcluster)  [unwired: 12 in, 3 out]
        n181 = Empty String/Path?(string/path=w516) -> (empty?=w517:bool)
        n182 = Path to Array of Strings(0:w516) -> (2:w520:string[])  [unwired: 1 out]
        n183 = Select(t=w510, s=w517, f=w516) -> (s? t:f=w515:path)
        n184 = Reverse 1D Array(array=w520) -> (reversed array=w519:string[])
        n185 = Index Array(array=w519) -> (element=w518:string)  [unwired: 1 in]
        n186 = call "File Dialog"("start path"=w515, "default name"=w518, "error in"=w511, "pattern (all files)"="*.gscript") -> ("selected path"=w524:path, "cancelled"=w521:bool, "error out"=w523:errorcluster)  [unwired: 8 in, 1 out]
        n187 = case shown="False" w521 {
          tunnel: w524 -> [_ w530]
          tunnel: w523 -> [_ w538]
          tunnel: [errorcluster {"status"=FALSE, "code"=0, "source"=""} ("error out") w531] -> w522
          frame True {
          }
          frame False {
            n188 = Open/Create/Replace File(file path (use dialog)=w530, error in=w538, access (0:read/write)=enum16{"read/write", "read-only", "write-only"}."read-only") -> (refnum out=w536:refnum<file>, error out=w535:errorcluster)  [unwired: 3 in, 1 out]
            n189 = local write "Script Path"(w530) -> ()
            n190 = Read from Text File(file (use dialog)=w536, error in=w535) -> (refnum out=w533:refnum<file>, text=w534:string, error out=w532:errorcluster)  [unwired: 2 in, 1 out]
            n191 = Close File(refnum=w533, error in=w532) -> (error out=w531:errorcluster)  [unwired: 1 out]
            n192 = local write "Script Input"(w534) -> ()
          }
        }
      }
      frame "Save Script", "Quicksave" {
        n193 = local read "Script Path"() -> (w546:path)
        n194 = call "Application Paths.vi"("gScript Interpreter in"=w543, "error in (no error)"=w541) -> ("gScript Interpreter out"=w542:refnum<class "gScript Interpreter.lvclass">, "Scripts Path"=w539:path, "error out"=w540:errorcluster)  [unwired: 12 in, 3 out]
        n195 = Empty String/Path?(string/path=w546) -> (empty?=w547:bool)
        n196 = Path to Array of Strings(0:w546) -> (2:w549:string[])  [unwired: 1 out]
        n197 = Select(t=w539, s=w547, f=w546) -> (s? t:f=w545:path)
        n198 = Reverse 1D Array(array=w549) -> (reversed array=w548:string[])
        n199 = Index Array(array=w548) -> (element=w544:string)  [unwired: 1 in]
        n200 = case shown="\"Save Script\"" w552 {
          tunnel: w540 -> [w561 w568]
          tunnel: [w560 w566] -> w555
          tunnel: [w561 w565] -> w554
          tunnel: [w559 w564] -> w553
          tunnel: w545 -> [w560 w563]
          tunnel: w544 -> [_ w562]
          frame "Quicksave", Default {
            n201 = Empty String/Path?(string/path=w560) -> (empty?=w559:bool)
          }
          frame "Save Script" {
            n202 = call "File Dialog3"("start path"=w563, "default name"=w562, "error in"=w568, "pattern (all files)"="*.gscript") -> ("selected path"=w566:path, "cancelled"=w564:bool, "error out"=w565:errorcluster)  [unwired: 8 in, 1 out]
          }
        }
        n203 = case shown="False" w553 {
          tunnel: [errorcluster {"status"=FALSE, "code"=0, "source"=""} ("error out") w573] -> w556
          tunnel: w555 -> [_ w571]
          tunnel: w554 -> [_ w580]
          tunnel: w551 -> [w569 w575]
          tunnel: [w569 w574] -> w550
          frame True {
          }
          frame False {
            n204 = Open/Create/Replace File(file path (use dialog)=w571, error in=w580, operation (0:open)=T13."replace or create", access (0:read/write)=enum16{"read/write", "read-only", "write-only"}."write-only") -> (refnum out=w584:refnum<file>, error out=w583:errorcluster)  [unwired: 2 in, 1 out]
            n205 = local read "Script Input"() -> (w579:string)
            n206 = Write to Text File(file (use dialog)=w584, text=w579, error in=w583) -> (refnum out=w582:refnum<file>, error out=w581:errorcluster)  [unwired: 1 in, 1 out]
            n207 = Close File(refnum=w582, error in=w581) -> (error out=w577:errorcluster)  [unwired: 1 out]
            n208 = Format Into String(format string="Saved script to %s", w571) -> (resulting string=w576:string)  [unwired: 2 in, 1 out]
            n209 = call "Add Line.vi"("error in"=w577, "String"=w576, "Console Log in"=w575) -> ("error out"=w573:errorcluster, "Console Log out"=w574:refnum<class "Console Log.lvclass">)  [unwired: 7 in]
            n210 = local write "Script Path"(w571) -> ()
          }
        }
      }
      frame "Load Project" {
        # "Steps\n  1. Get New path from user.\n  2. Replace path in config file with new value\n  3. Destroy the Gantry object\n  4. Reset interpreter object\n  5. Initialize"
        n211 = call "Find Project Folder.vi"("error in (no error)"=w595, "overwrite"=TRUE, "gScript Interpreter in"=w597) -> ("error out"=w586:errorcluster, "gScript Interpreter out"=w593:refnum<class "gScript Interpreter.lvclass">)  [unwired: 7 in]
        n212 = case shown="No Error" w586 {
          selector: w586 -> [w606 w635]
          tunnel: w593 -> [w622 w637]
          tunnel: w592 -> [w617 w638]
          tunnel: [w614 w638] -> w591
          tunnel: [w603 w636] -> w590
          tunnel: [w612 w637] -> w589
          tunnel: [w602 w635] -> w588
          tunnel: w587 -> [w611 w636]
          frame No Error {
            # "Save copy of Aerotech Controller Ref to use\nAsynchronously with ESTOP"
            n213 = call "Reset Interpreter.vi"("error in (no error)"=w606, "gScript Interpreter in"=w622) -> ("error out"=w610:errorcluster, "gScript Interpreter out"=w616:refnum<class "gScript Interpreter.lvclass">)  [unwired: 8 in]
            n214 = call-dynamic "Read Virtual Mode.vi"("error in (no error)"=w610, "Gantry in"=w611) -> ("error out"=w609:errorcluster, "Virtual Mode"=w599:T1, "Gantry out"=w608:refnum<class "Gantry.lvclass">)  [unwired: 6 in, 1 out]
            n215 = call "Destroy.vi"("error in"=w609, "Gantry Class in"=w608) -> ("error out"=w615:errorcluster)  [unwired: 9 in]
            n216 = control-ref of="Script Input"() -> (w613:refnum<vi>)
            n217 = call "Highlight Line.vi"("error in (no error)"=w615, "Line Number"=-1, "String Field In"=w613) -> ("error out"=w619:errorcluster)  [unwired: 7 in, 1 out]
            n218 = call "Clear Console.vi"("error in (no error)"=w619, "Console Log in"=w617) -> ("error out"=w618:errorcluster, "Console Log out"=w620:refnum<class "Console Log.lvclass">)  [unwired: 8 in]
            n219 = call "Initialize Gantry.vi"("Console Log in"=w620, "error in (no error)"=w618, "Virtual Mode"=w599, "Prompt for Virtual Mode"=FALSE, "gScript Interpreter in"=w616) -> ("error out"=w604:errorcluster, "Gantry out"=w605:refnum<class "Gantry.lvclass">, "gScript Interpreter out"=w612:refnum<class "gScript Interpreter.lvclass">, "Console Log out"=w614:refnum<class "Console Log.lvclass">)  [unwired: 3 in]
            n220 = disable-structure shown="GANTRY_DRIVER==AUTOMATION1" {
              disable-tunnel: w605 -> [w628 w634]
              disable-tunnel: w604 -> [w627 w633]
              disable-tunnel: [w626 w632] -> w603
              disable-tunnel: [w625 w631] -> w602
              disable-tunnel: [w623 w629] -> w598
              frame condition #0 {
                n221 = call "Read Gantry Controller A3200.vi"("error in (no error)"=w627, "Gantry in"=w628) -> ("error out"=w625:errorcluster, "A3200 controller out"=w624:refnum<k24>, "Gantry out"=w626:refnum<class "Gantry.lvclass">)  [unwired: 7 in]
                n222 = To Variant(anything=w624) -> (Variant=w623:variant)
              }
              frame condition #1 (active) {
                n223 = call "Read Gantry Controller AUTOMATION1.vi"("error in (no error)"=w633, "Gantry in"=w634) -> ("error out"=w631:errorcluster, "Controller AUTOMATION1"=w630:refnum<k24>, "Gantry out"=w632:refnum<class "Gantry.lvclass">)  [unwired: 7 in]
                n224 = To Variant(anything=w630) -> (Variant=w629:variant)
              }
            }
            n225 = Bundle By Name(cluster=T2 {"Controller Ref"=variant, "Virtual Mode"=enum."Nonvirtual"} ("Aerotech controller Ref"), "Controller Ref"=w598, "Virtual Mode"=w599) -> (w601:T2)
            n226 = local write "Aerotech controller Ref"(w601) -> ()
          }
          frame Error {
          }
        }
      }
      frame "Exit" {
        n227 = call "Destroy.vi"("error in"=w642, "Gantry Class in"=w641) -> ("error out"=w640:errorcluster)  [unwired: 9 in]
      }
    }
    n228 = call <vilib>:"Clear Errors.vi"("error in (no error)"=w295) -> ("error out"=w297:errorcluster)  [unwired: 5 in, 1 out]
  }
  n229 = Release Queue(queue=w10) -> ()  [unwired: 2 in, 3 out]
  n230 = call "Destroy.vi"("error in"=w8, "Console Log in"=w16) -> ()  [unwired: 9 in, 1 out]
